vi "Test Cases - timestamp.vi"() -> ()   [LabVIEW 2017]
uses:
  API-String-Arugments-Support/API String Arguments Support.lvlib
panel:
  in  "UTC? (F)":bool=TRUE
  out "String 4":string="2023-10-31T14:49:39.597Z"
  in  "Time Stamp 4":timestamp=timestamp(3781608579.597416 s since 1904-01-01)
  out "Timestamp 4'":timestamp
  out "String 3":string="2023-10-31T14:49:39.597Z"
  out "data 3":timestamp=timestamp(3779880873 s since 1904-01-01)
  out "data 2":timestamp=timestamp(3781608579.597 s since 1904-01-01)
  out "Timestamp 1'":timestamp=timestamp(3781608579.597 s since 1904-01-01)
  out "concatenated string":string="2023-10-11 22:54:33(%<%Y-%m-%d %H:%M:%S>T)"
  out "error 3":errorcluster
  out "error 2":errorcluster
  in  "String 2":string="2023-10-31T14:49:39.597Z"
  in  "Time Stamp 3":timestamp=timestamp(3779880873.3011937 s since 1904-01-01)
  out "error":errorcluster
  in  "Time Stamp 1":timestamp=timestamp(3781608579.597416 s since 1904-01-01)
  out "String":string="2023-10-31T14:49:39.597Z"
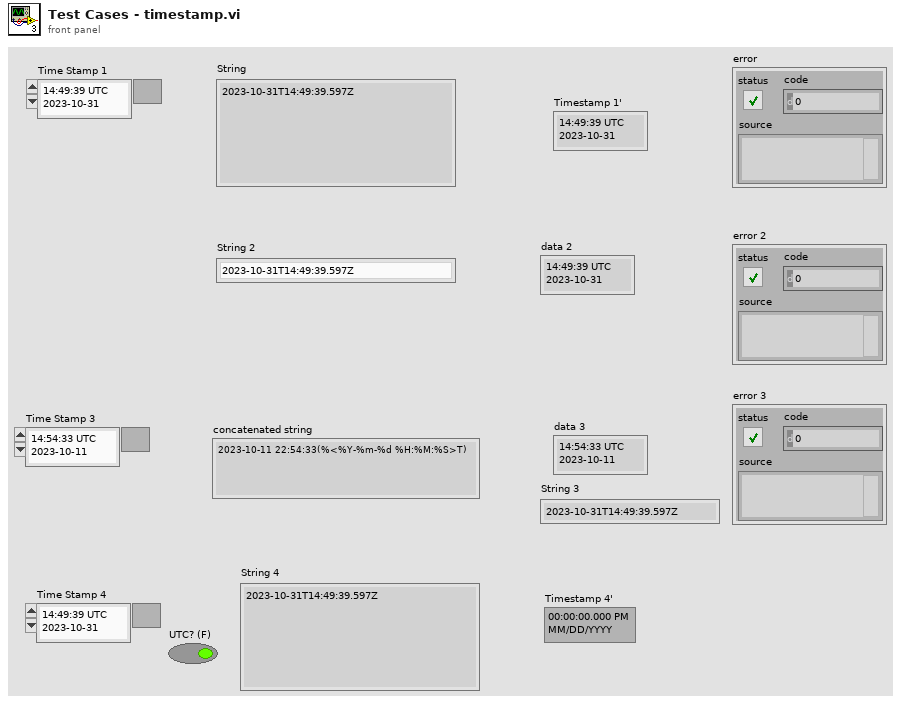
[diagram p1: front panel]
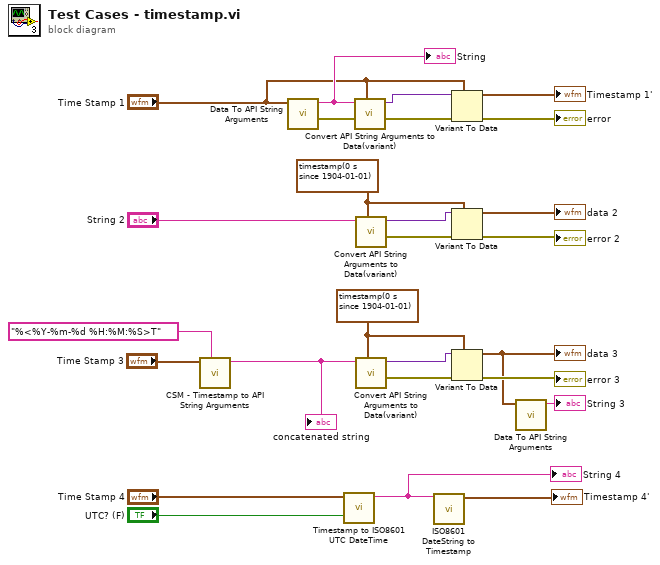
[diagram p0: block diagram]
diagram:
  w17 = timestamp(0 s since 1904-01-01) ("Time Stamp")
  w14 = timestamp(0 s since 1904-01-01) ("Time Stamp")
  n1 = call "CSM - Timestamp to API String Arguments.vi"("Format(Empty to use UTC)"="%<%Y-%m-%d %H:%M:%S>T" ("format string"), "Timestamp (now)"="Time Stamp 3") -> ("CSM Timestamp Argument"=w1:string)  [unwired: 9 in]
  "concatenated string" <- w1
  n2 = call "Data To API String Arguments.vi"("data"="Time Stamp 1") -> ("error out"=w25:errorcluster, "String"=w26:string)  [unwired: 9 in]
  "String" <- w26
  n3 = call <vilib>:"Timestamp to ISO8601 UTC DateTime.vi"("UTC? (F)"="UTC? (F)", "Timestamp (now)"="Time Stamp 4") -> ("ISO8601 UTC DateTime"=w5:string)  [unwired: 9 in]
  "String 4" <- w5
  n4 = call "Convert API String Arguments to Data(variant).vi"("Type"="Time Stamp 1", "error in (no error)"=w25, "String"=w26) -> ("error"=w24:errorcluster, "Data"=w12:variant)  [unwired: 7 in]
  n5 = call "Convert API String Arguments to Data(variant).vi"("Type"=w14, "String"="String 2") -> ("error"=w22:errorcluster, "Data"=w15:variant)  [unwired: 8 in]
  n6 = call "Convert API String Arguments to Data(variant).vi"("Type"=w17, "String"=w1) -> ("error"=w21:errorcluster, "Data"=w16:variant)  [unwired: 8 in]
  n7 = call <vilib>:"ISO8601 DateString to Timestamp.vi"("ISO8601 Date String"=w5) -> ("Timestamp"=→"Timestamp 4'":timestamp)  [unwired: 8 in, 2 out]
  n8 = Variant To Data(error in=w24, type="Time Stamp 1", Variant=w12) -> (data=→"Timestamp 1'":timestamp, error out=→"error":errorcluster)
  n9 = Variant To Data(error in=w22, type=w14, Variant=w15) -> (data=→"data 2":timestamp, error out=→"error 2":errorcluster)
  n10 = Variant To Data(error in=w21, type=w17, Variant=w16) -> (data=w9:timestamp, error out=→"error 3":errorcluster)
  "data 3" <- w9
  n11 = call "Data To API String Arguments.vi"("data"=w9) -> ("String"=→"String 3":string)  [unwired: 9 in, 1 out]
